vi "Write.vi"(8 "error in (no error)":errorcluster, 10 "DATA":T1, 11 "With Data in":refnum<class "With Data.lvclass">) -> (0 "error out":errorcluster, 3 "With Data out":refnum<class "With Data.lvclass">)   [LabVIEW 2020, in "With Data.lvclass"]
uses:
  With Data.lvclass
  With Data.lvclass/With Data.ctl
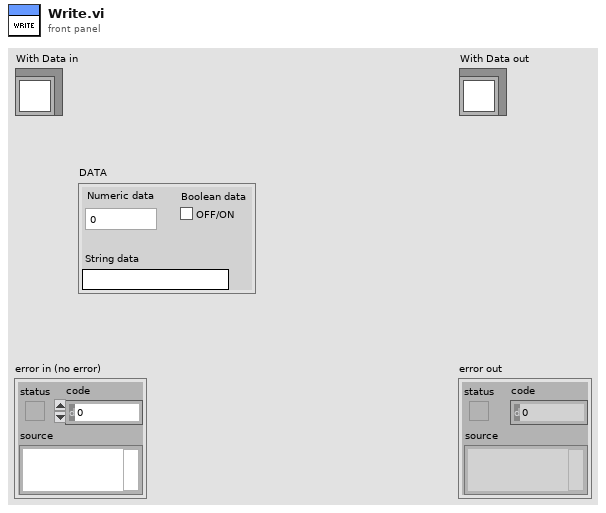
[diagram p1: front panel]
types:
  T1 = cluster{"Numeric data":dbl, "String data":string, "Boolean data":bool}
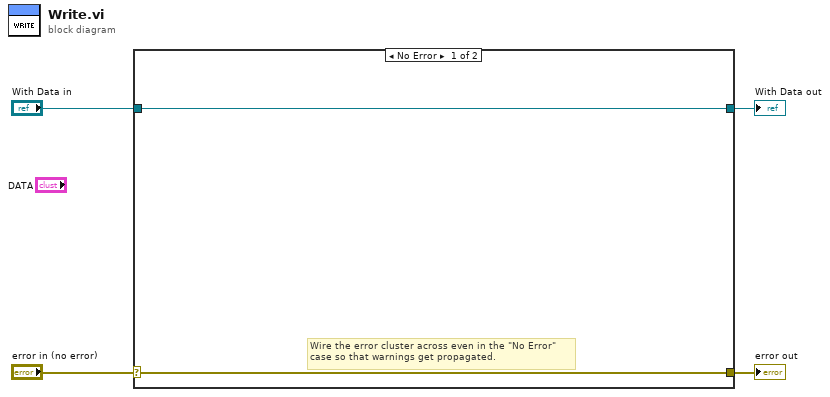
[diagram p0: block diagram]
diagram:
  n1 = case shown="No Error" "error in (no error)" {
    selector: "error in (no error)" -> [w6 w8]
    tunnel: [w6 w8] -> w3
    tunnel: [w5 w7] -> w1
    tunnel: "With Data in" -> [w5 w7]
    frame No Error {
      # "Wire the error cluster across even in the \"No Error\"\ncase so that warnings get propagated."
    }
    frame Error {
    }
  }
  "error out" <- w3
  "With Data out" <- w1
